vi "Noise-Buffer.vi"(2 "Action":T1(ring), 5 "Npts":i32, 7 "Data In":dbl[](array[numeric]), 9 "Name":string, 11 "error in (no error)":errorcluster) -> (8 "Data Out":dbl[](array[numeric]), 15 "error out":errorcluster)   [LabVIEW 2020]
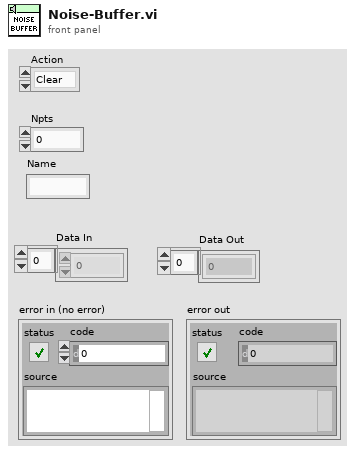
[diagram p1: front panel]
types:
  T1 = enum16{"Clear", "Set data", "Reset index", "Get data"}
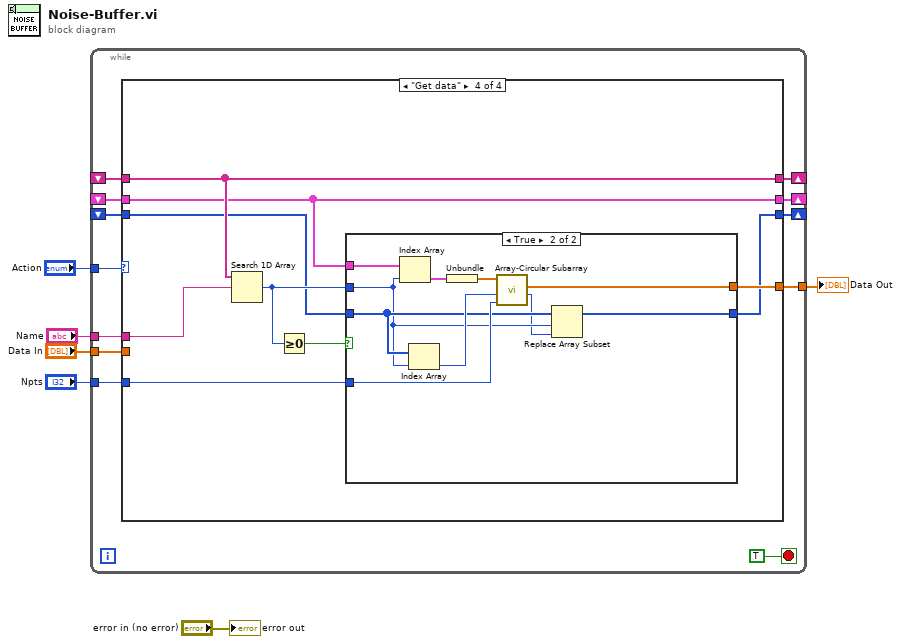
[diagram p0: block diagram]
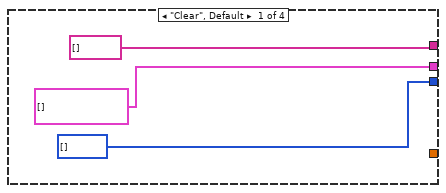
[diagram p2: hidden frame]
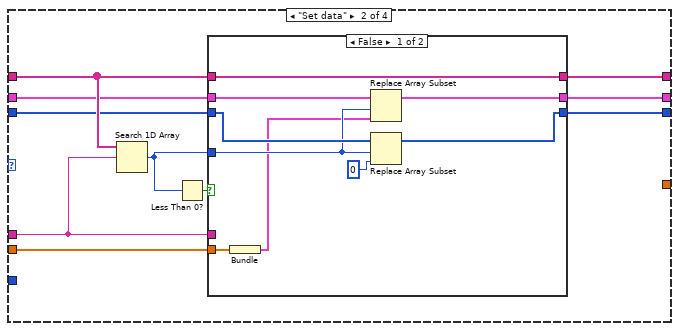
[diagram p3: hidden frame]
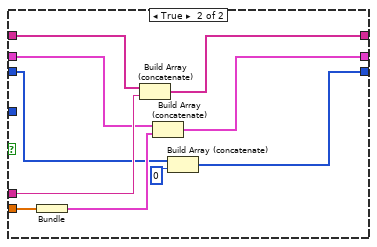
[diagram p4: hidden frame]
diagram:
  n1 = while {
    shift-right: [w17] -> _
    shift-left: _ -> [w16]
    shift-right: [w15] -> _
    shift-left: _ -> [w14]
    tunnel: "Action" -> [w13]
    shift-right: [w12] -> _
    shift-left: _ -> [w11]
    tunnel: "Name" -> [w10]
    tunnel: "Data In" -> [w9]
    tunnel: "Npts" -> [w8]
    tunnel: [w7] -> w2
    stop <- TRUE stop-if-true
    n2 = case shown="\"Get data\"" w13 {
      tunnel: [string[] [] w25 w53 w61] -> w17
      tunnel: w16 -> [_ w30 w53 w61]
      tunnel: [cluster{dbl[]}[] [] w24 w52 w59] -> w15
      tunnel: w14 -> [_ w29 w52 w59]
      tunnel: [i32[] [] w23 w51 w54] -> w12
      tunnel: w11 -> [_ w28 w51 w56]
      tunnel: w10 -> [_ w26 _ w62]
      tunnel: w9 -> [_ w27 _ _]
      tunnel: w8 -> [_ _ _ w57]
      tunnel: [_ _ _ w55] -> w7
      frame "Clear", Default {
      }
      frame "Set data" {
        n3 = Search 1D Array(1D array=w30, element=w26) -> (index of element=w22:i32)  [unwired: 1 in]
        n4 = Less Than 0?(x=w22) -> (x < 0?=w31:bool)
        n5 = case shown="False" w31 {
          tunnel: w30 -> [w40 w50]
          tunnel: w29 -> [w36 w45]
          tunnel: w28 -> [w39 w43]
          tunnel: w27 -> [w33 w47]
          tunnel: w26 -> [_ w49]
          tunnel: [w40 w48] -> w25
          tunnel: [w35 w44] -> w24
          tunnel: [w37 w41] -> w23
          tunnel: w22 -> [w34 _]
          frame False {
            n6 = Bundle("Data In"=w33) -> (w32:cluster{"Data In":dbl[]})  [unwired: 1 in]
            n7 = Replace Array Subset(array=w36, new element=w32, index=w34) -> (w35:cluster{"Data In":dbl[]}[])
            n8 = Replace Array Subset(array=w39, new element=0 ("new element/subarray"), index=w34) -> (w37:i32[])
          }
          frame True {
            n9 = Bundle("Data In"=w47) -> (w46:cluster{"Data In":dbl[]})  [unwired: 1 in]
            n10 = Build Array (concatenate)(w50, w49) -> (w48:string[])
            n11 = Build Array (concatenate)(w45, w46) -> (w44:cluster{"Data In":dbl[]}[])
            n12 = Build Array (concatenate)(w43, 0) -> (w41:i32[])
          }
        }
      }
      frame "Reset index" {
      }
      frame "Get data" {
        n13 = Search 1D Array(1D array=w61, element=w62) -> (index of element=w58:i32)  [unwired: 1 in]
        n14 = Greater Or Equal To 0?(x=w58) -> (x >= 0?=w60:bool)
        n15 = case shown="True" w60 {
          tunnel: w59 -> [_ w73]
          tunnel: w58 -> [_ w66]
          tunnel: w57 -> [_ w70]
          tunnel: w56 -> [w63 w67]
          tunnel: [_ w68] -> w55
          tunnel: [w63 w64] -> w54
          frame False {
          }
          frame True {
            n16 = Index Array(array=w73, index=w66) -> (element=w72:cluster{"Data In":dbl[]})
            n17 = Index Array(array=w67, index=w66) -> (element=w69:i32)
            n18 = Unbundle(w72) -> ("Data In"=w71:dbl[])
            n19 = call "Array-Circular Subarray.vi"("Npts"=w70, "Offset (in)"=w69, "Array"=w71) -> ("Offset (out)"=w65:i32, "Subarray"=w68:dbl[])  [unwired: 7 in]
            n20 = Replace Array Subset(array=w67, new element=w65, index=w66) -> (w64:i32[])
          }
        }
      }
    }
  }
  "Data Out" <- w2
  "error out" <- "error in (no error)"
